vi "Choreo_TrajectorySwerve_Splits.vi"(11 "ChoreoTrajectorySwerve":T1) -> (3 "splits":i32[](array[numeric]))   [LabVIEW 2019, in "ChoreoLib.lvlib"]
doc: "Create an empty trajectory\n\nInputs: \n <none>\n\nOutputs:\n - ChoreoTrajectory - array - Empty array of Trajectory states."
uses:
  ChoreoLib.lvlib
  TypeDef/ChoreoSwerveSample.ctl
  TypeDef/ChoreoEventMarker.ctl
  TypeDef/ChoreoTrajectorySwerve.ctl
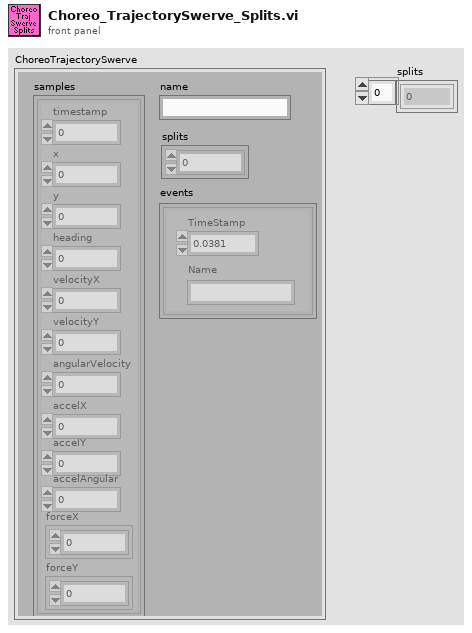
[diagram p1: front panel]
types:
  T1 = typedef "ChoreoLib.lvlib/ChoreoTrajectorySwerve.ctl" = cluster{"name":string, "samples":T2[], "splits":i32[], "events":T3[]}
  T2 = typedef "ChoreoLib.lvlib/ChoreoSwerveSample.ctl" = cluster{"timestamp":dbl, "x":dbl, "y":dbl, "heading":dbl, "velocityX":dbl, "velocityY":dbl, "angularVelocity":dbl, "accelX":dbl, "accelY":dbl, "accelAngular":dbl, "forceX":dbl[], "forceY":dbl[]}
  T3 = typedef "ChoreoLib.lvlib/ChoreoEventMarker.ctl" = cluster{"TimeStamp":dbl, "Name":string}
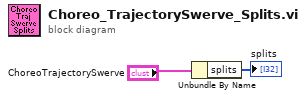
[diagram p0: block diagram]
diagram:
  n1 = Unbundle By Name("ChoreoTrajectorySwerve") -> ("splits"=→"splits":i32[])
